vi "labview_robotjoint_states_Server.vi"() -> ()   [LabVIEW 2013]
doc: "Template server that runs individual ros topics, services, etc. This is cloned for each topic being run."
uses:
  SubVIs/_ROSControl.ctl
  SubVIs/_ROSDirection.ctl
  _ROSDefinition.vi
panel:
  out "Init Count":i32
  out "queue":string
  out "Connected":bool
  out "str to write":string
  out "Status":T1(ring) caption="Connected?"
  out "Specs":T3={"Server"="", "Node"="/labview", "Server Port"=5000, "URI (Subsc)"="", "Direction"=enum."Node"}
  out "Service Reply":string
  out "unregister":string="<?xml version='1.0'?>\n<methodResponse>\n<params>\n<param>\n<value><array><data>\n<value><int>1</int></value>\n<value><string>Registered [/labview] as publisher of [/robot/head/command_head_nod]</string></value>\n<value><array><data>\n<value><string>http://tuftsBaxter.local:56995/</string></value>\n</data></array></value>\n</data></array></value>\n</param>\n</params>\n</methodResponse>\n"
  out "Requests":T4(array[cluster])
  out "Last Reply":string
  in  "stop":bool
  out "error out":errorcluster
  out "Connections":T5(array[cluster])
  in  "Baxter":T6
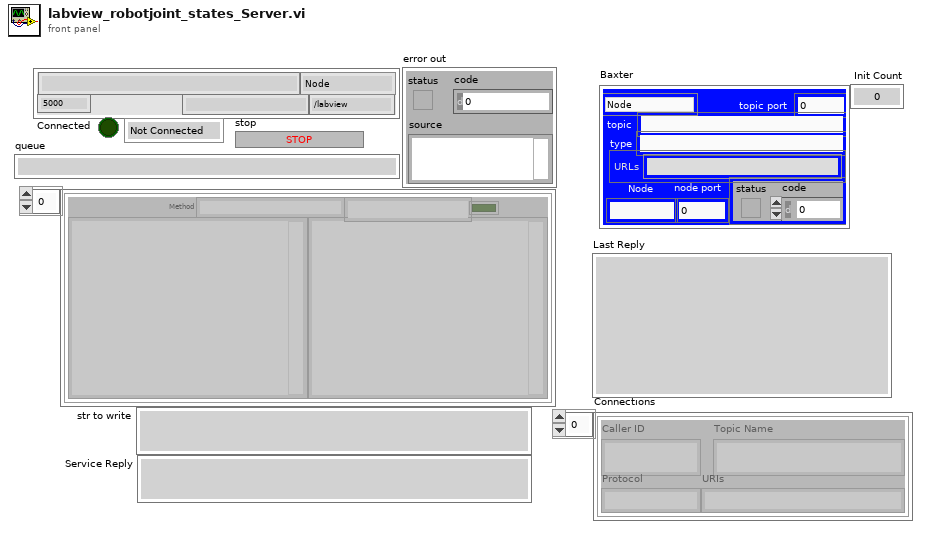
[diagram p1: front panel]
types:
  T1 = enum16{"Not Connected", "Registered", "Connected"}
  T2 = typedef "_ROSDirection.ctl" = enum16{"Node", "Publisher", "Subscriber", "Service Client"}
  T3 = cluster{"Server":string, "Node":string, "Server Port":u32, "URI (Subsc)":string, "Direction":T2}
  T4 = cluster{"First":string, "Second":string, "Method":string, "success":bool, "Dir1":string, "Dir2":string, "time":string}[]
  T5 = cluster{"Caller ID":string, "Topic Name":string, "Protocol":string, "URIs":string}[]
  T6 = typedef "_ROSControl.ctl" = cluster{"topic port":u16, "Node":string, "topic":string, "type":string, "node port":u32, "error ":errorcluster, "Direction":T2, "APIs":string[]}
  T7 = cluster{"data out":string, "data out 2":string, "data out 3":string, "Success?":bool, "data out 4":string, "data out 5":string, "time":string}[]
  T8 = cluster{"Code":i32, "Status Message":string, "APIs":string[]}
  T9 = cluster{"Server":string, "Node":string, "Server Port":u32, "URI (Subsc)":string, "connection":refnum<k5>, "Direction":T2}
  T10 = cluster{"Caller ID":string, "Topic Name":string, "Protocol":string, "URIs":string}
  T11 = cluster{string, "data out":string, "Node":string, bool, string, string, "Current Time":string}
  T12 = cluster{string, string, string, bool, string, string, "Current Time":string}
  T13 = cluster{"Protocol":string, "Code":i32, "IP":string, "Port":i32}
  T14 = cluster{"Node":string, "topic":string, "topic":string, "topic":string}
  T15 = cluster{"Code":i8, "statusMessage":string, "APIs":string[]}
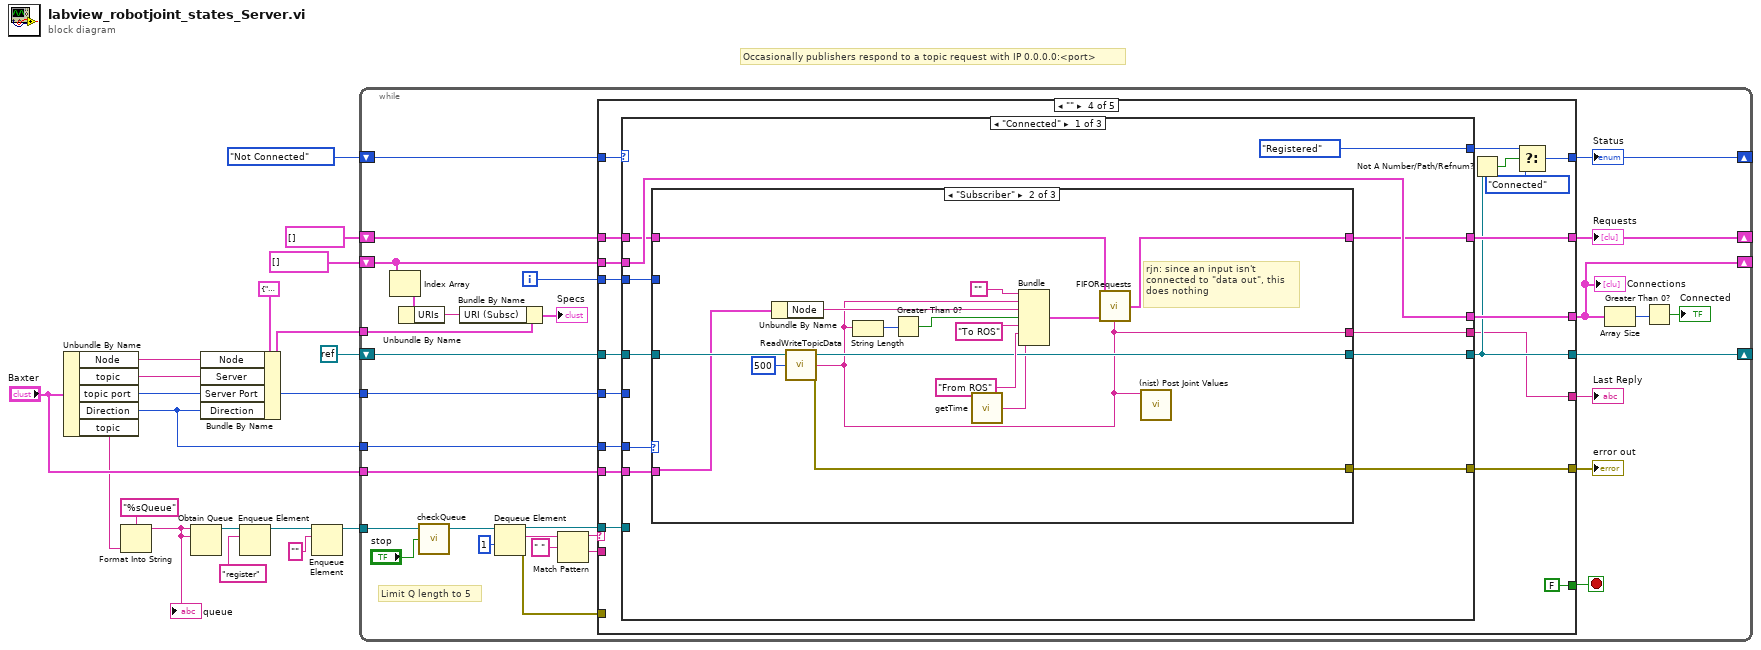
[diagram p0: block diagram]
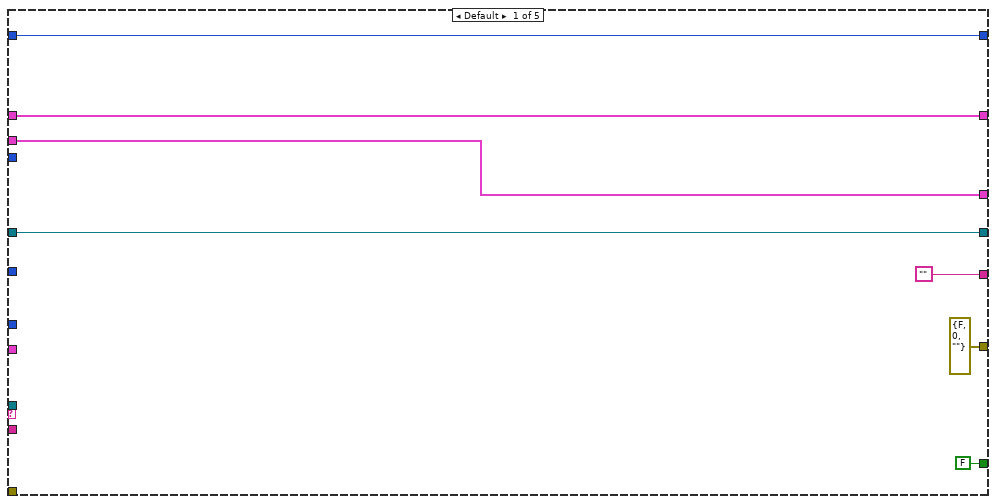
[diagram p2: hidden frame]
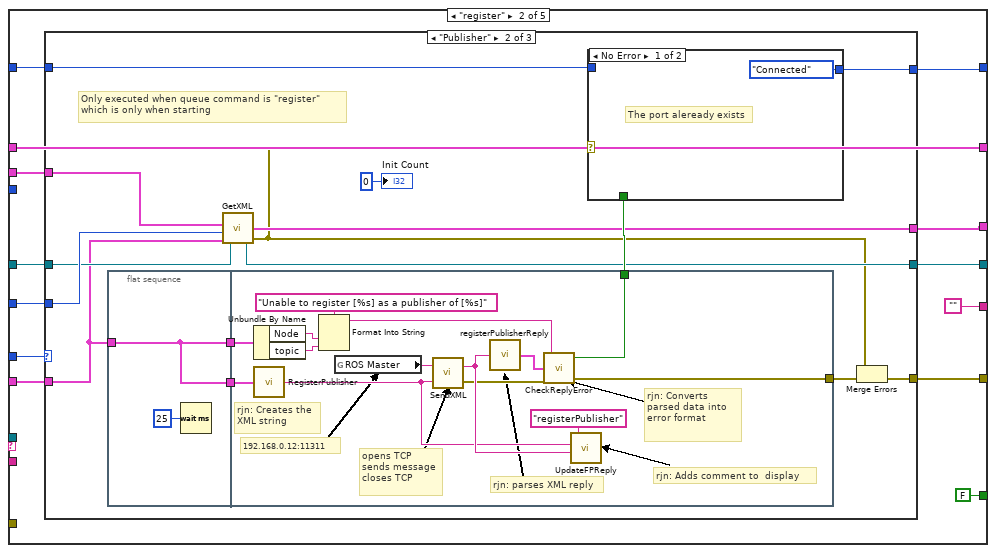
[diagram p3: hidden frame]
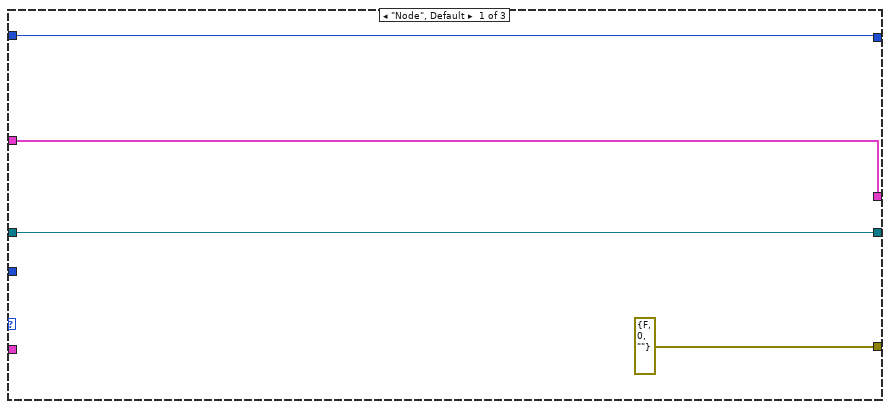
[diagram p4: hidden frame]
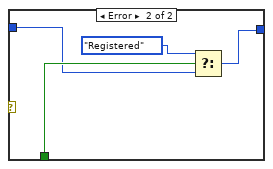
[diagram p5: hidden frame]
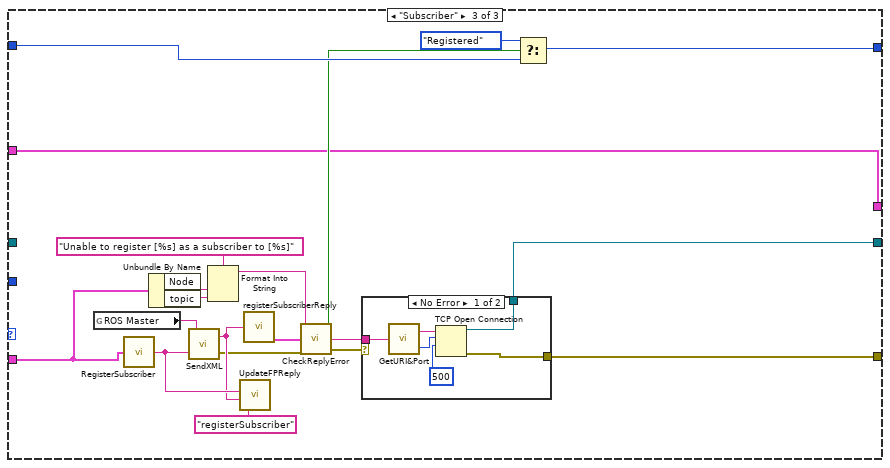
[diagram p6: hidden frame]
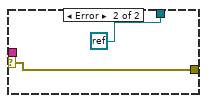
[diagram p7: hidden frame]
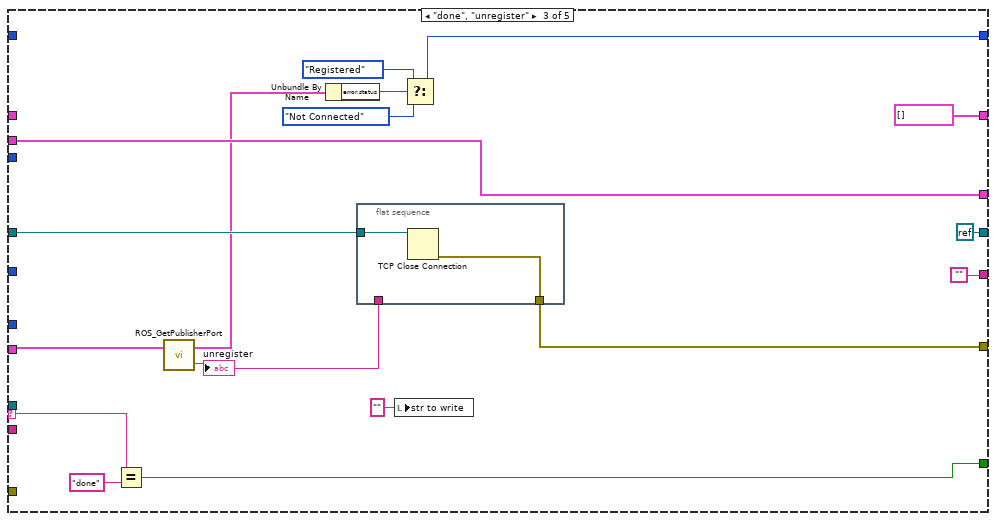
[diagram p8: hidden frame]
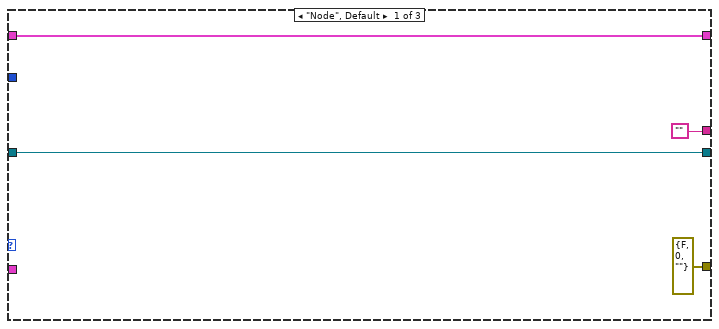
[diagram p9: hidden frame]
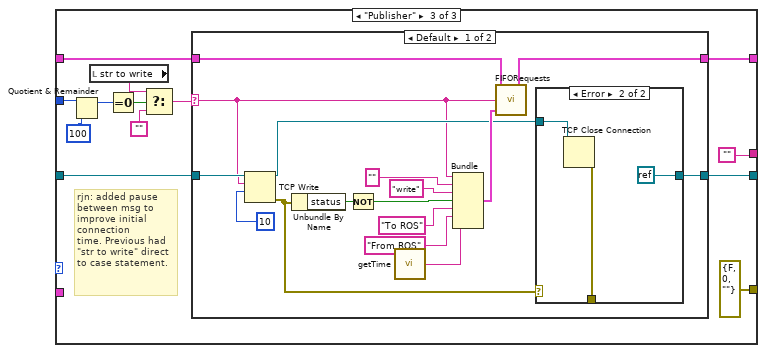
[diagram p10: hidden frame]
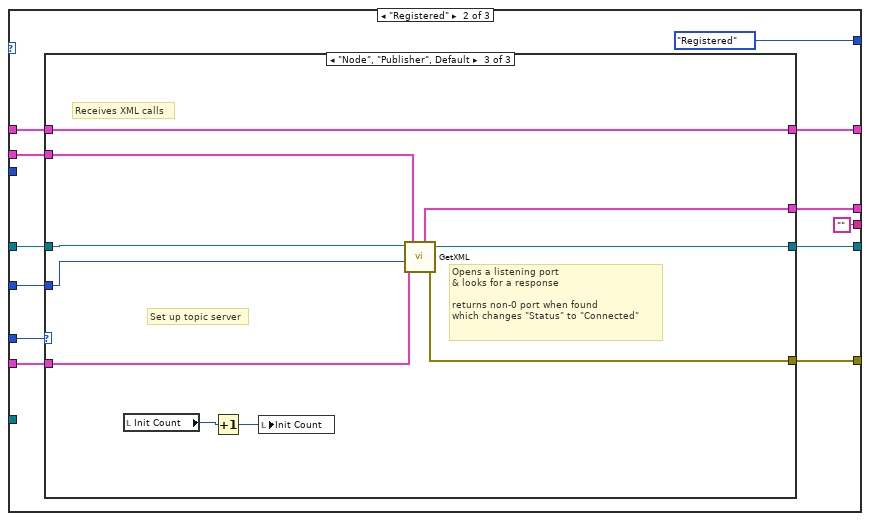
[diagram p13: hidden frame]
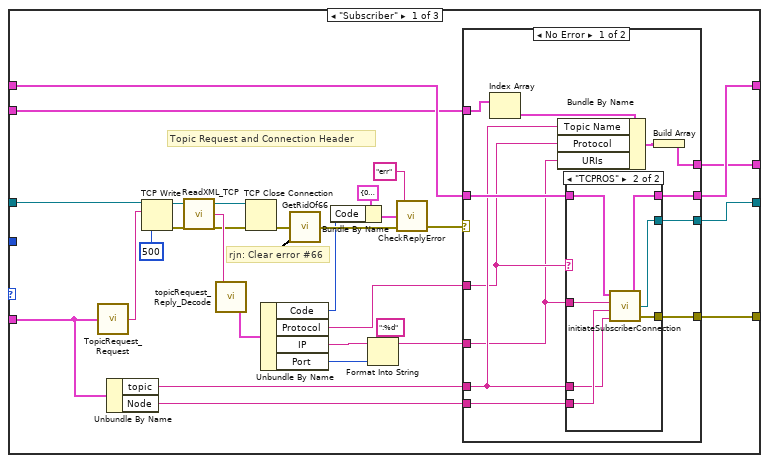
[diagram p14: hidden frame]
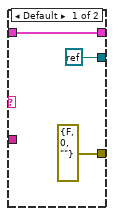
[diagram p15: hidden frame]
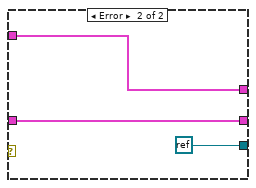
[diagram p16: hidden frame]
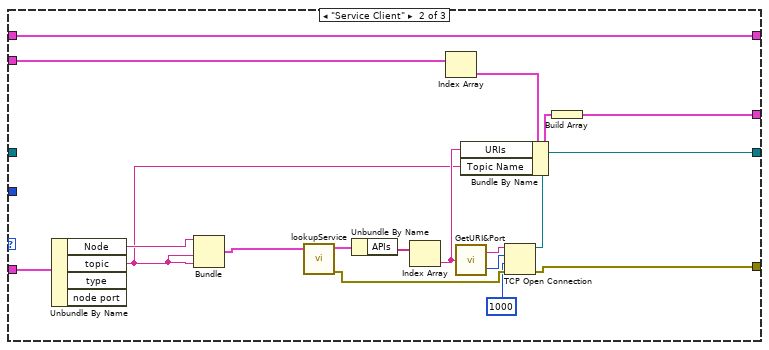
[diagram p17: hidden frame]
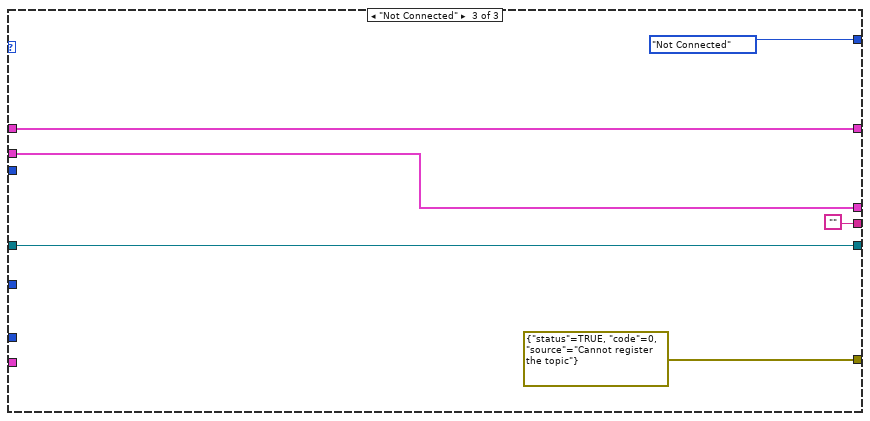
[diagram p18: hidden frame]
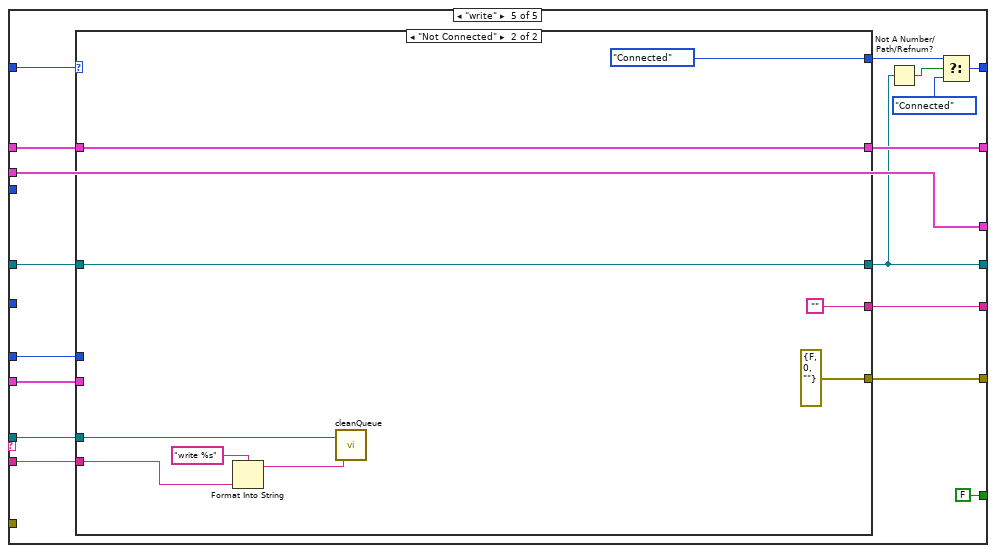
[diagram p19: hidden frame]
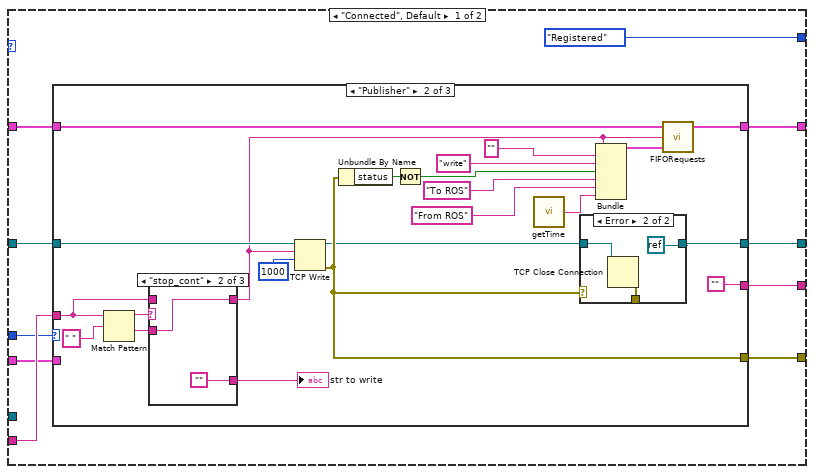
[diagram p20: hidden frame]
diagram:
  # "Occasionally publishers respond to a topic request with IP 0.0.0.0:<port>"
  n1 = Unbundle By Name("Baxter") -> ("Node"=w4:string, "topic"=w3:string, "topic port"=w1:u16, "Direction"=w2:T2, "topic"=w9:string)
  n2 = Format Into String(format string="%sQueue", w9) -> (resulting string=w18:string)  [unwired: 2 in, 1 out]
  "queue" <- w18
  n3 = Obtain Queue(name (unnamed)=w18, element data type=w18) -> (queue out=w12:refnum<queue>)  [unwired: 3 in, 2 out]
  n4 = Bundle By Name(cluster=T3 {"Server"="", "Node"="/labview", "Server Port"=5000, "URI (Subsc)"="", "Direction"=enum."Node"} ("Specs"), "Node"=w4, "Server"=w3, "Server Port"=w1, "Direction"=w2) -> (w10:T3)
  n5 = Enqueue Element(queue=w12, element="register") -> (queue out=w7:refnum<queue>)  [unwired: 2 in, 2 out]
  n6 = Enqueue Element(queue=w7, element="") -> (queue out=w6:refnum<queue>)  [unwired: 2 in, 2 out]
  n7 = while {
    tunnel: w1 -> [w50]
    shift-right: [w25] -> _
    shift-left: T5 [] ("Connections") -> [w34]
    shift-right: [w39] -> _
    shift-left: refnum<k0> refnum -> [w48]
    tunnel: w2 -> [w49]
    tunnel: "Baxter" -> [w47]
    shift-right: [w40] -> _
    shift-left: T7 [] ("Requests In") -> [w41]
    shift-right: [w36] -> _
    shift-left: T1."Not Connected" ("Status") -> [w37]
    tunnel: w10 -> [w32]
    tunnel: w6 -> [w26]
    i -> [w21]
    stop <- w38 stop-if-true
    # "Limit Q length to 5"
    n8 = Index Array(array=w34) -> (element=w33:T10)  [unwired: 1 in]
    n9 = Unbundle By Name(w33) -> ("URIs"=w31:string)
    n10 = call "checkQueue.vi"("stop"="stop", "queue in"=w26) -> ("queue out"=w28:refnum<queue>)  [unwired: 3 in]
    n11 = Bundle By Name(cluster=w32, "URI (Subsc)"=w31) -> (→"Specs":T3)
    n12 = Dequeue Element(queue=w28, timeout in ms (-1)=1) -> (queue out=w29:refnum<queue>, element=w45:string, error out=w22:errorcluster)  [unwired: 1 in, 1 out]
    n13 = Match Pattern(string=w45, regular expression=" ") -> (before substring=w43:string, after substring=w42:string)  [unwired: 1 in, 2 out]
    n14 = case shown="\"\"" w43 {
      selector: w43 -> [_ _ w144 _ _]
      tunnel: w50 -> [_ w69 _ w176 _]
      tunnel: w34 -> [w57 w61 w154 w175 w360]
      tunnel: [w57 w60 w154 w174 w360] -> w25
      tunnel: w49 -> [_ w70 _ w173 w352]
      tunnel: [w56 w66 refnum<k0> refnum w167 w353] -> w39
      tunnel: w48 -> [w56 w65 w155 w168 w359]
      tunnel: w47 -> [_ w68 w153 w172 w350]
      tunnel: w42 -> [_ _ _ _ w357]
      tunnel: [FALSE FALSE w142 FALSE FALSE] -> w38
      tunnel: [errorcluster {"status"=FALSE, "code"=0, "source"=""} ("error out") w67 w147 w169 w354] -> w35
      tunnel: w41 -> [w55 w64 _ w171 w356]
      tunnel: [w55 w64 T7 [] ("Requests Out") w170 w355] -> w40
      tunnel: w37 -> [w54 w63 _ w161 w358]
      tunnel: [w54 w62 w149 w162 w345] -> w36
      tunnel: ["" "" "" w166 w351] -> w20
      tunnel: w29 -> [_ _ _ w165 w349]
      tunnel: w22 -> [_ _ _ _ _]
      tunnel: w21 -> [_ _ _ w158 _]
      frame Default {
      }
      frame "register" {
        n15 = case shown="\"Publisher\"" w70 {
          tunnel: w69 -> [_ w84 _]
          tunnel: w68 -> [_ w81 w121]
          tunnel: [errorcluster {"status"=FALSE, "code"=0, "source"=""} ("error IO") w79 w118] -> w67
          tunnel: [w74 w82 w119] -> w66
          tunnel: w65 -> [w74 w83 _]
          tunnel: w63 -> [w73 w88 w114]
          tunnel: [w73 w87 w112] -> w62
          tunnel: w61 -> [w72 w86 w111]
          tunnel: [w72 w85 w111] -> w60
          frame "Node", Default {
          }
          frame "Publisher" {
            # "Only executed when queue command is \"register\"\nwhich is only when starting"
            n16 = flat-sequence {
              tunnel: w81 -> [w90]
              tunnel: [w90] -> w77
              tunnel: [w90] -> w75
              tunnel: [w95] -> w89
              tunnel: [w93] -> w80
              tunnel: w77 -> [w94]
              tunnel: w75 -> [w92]
              frame #0 {
                n17 = Wait (ms)(milliseconds to wait=u32 25) -> ()  [unwired: 1 out]
              }
              frame #1 {
                # "rjn: Adds comment to  display"
                # "rjn: Converts parsed data into\nerror format"
                # "rjn: parses XML reply"
                # "192.168.0.12:11311"
                # "opens TCP\nsends message\ncloses TCP"
                # "rjn: Creates the \nXML string"
                n18 = Unbundle By Name(w94) -> ("Node"=w101:string, "topic"=w100:string)
                n19 = call "RegisterPublisher.vi"("ROS"=w92) -> ("XML"=w99:string)
                n20 = Format Into String(format string="Unable to register [%s] as a publisher of [%s]", w101, w100) -> (resulting string=w97:string)  [unwired: 2 in, 1 out]
                n21 = global read "_ROSDefinition.vi" "ROS Master"() -> (w105:string)
                n22 = call "SendXML.vi"("Send"=w99, "URI in"=w105) -> ("error out"=w96:errorcluster, "Reply"=w104:string)
                n23 = call "registerPublisherReply.vi"("Response"=w104) -> ("Response"=w98:T8)
                n24 = call "CheckReplyError.vi"("error in"=w96, "Response"=w98, "Error String"=w97) -> ("error out"=w93:errorcluster, "Registered?"=w95:bool)  [unwired: 1 out]
                n25 = call "UpdateFPReply.vi"("Reply"=w104, "Sent"=w99, "method"="registerPublisher") -> ()  [unwired: 3 in]
              }
            }
            n26 = call "GetXML.vi"("Baxter"=w81, "topic port"=w84, "Connections"=w86, "connection ID in"=w83) -> ("error IO"=w78:errorcluster, "Subscribers"=w85:T5, "connection ID out"=w82:refnum<k5>)
            n27 = case shown="No Error" w78 {
              tunnel: w89 -> [_ w110]
              tunnel: w88 -> [_ w109]
              tunnel: [T1."Connected" ("f") w107] -> w87
              frame No Error {
                # "The port aleready exists"
              }
              frame Error {
                n28 = Select(t=T1."Registered", s=w110, f=w109) -> (s? t:f=w107:T1)
              }
            }
            n29 = Merge Errors(w78, w80) -> (w79:errorcluster)
            "Init Count" <- 0
          }
          frame "Subscriber" {
            n30 = global read "_ROSDefinition.vi" "ROS Master"() -> (w130:string)
            n31 = call "RegisterSubscriber.vi"("ROS"=w121) -> ("XML"=w128:string)
            n32 = Unbundle By Name(w121) -> ("Node"=w125:string, "topic"=w124:string)
            n33 = call "SendXML.vi"("Send"=w128, "URI in"=w130) -> ("error out"=w117:errorcluster, "Reply"=w127:string)
            n34 = Format Into String(format string="Unable to register [%s] as a subscriber to [%s]", w125, w124) -> (resulting string=w122:string)  [unwired: 2 in, 1 out]
            n35 = call "UpdateFPReply.vi"("Reply"=w127, "Sent"=w128, "method"="registerSubscriber") -> ()  [unwired: 3 in]
            n36 = call "registerSubscriberReply.vi"("Response"=w127) -> ("Response"=w126:T8)
            n37 = call "CheckReplyError.vi"("error in"=w117, "Response"=w126, "Error String"=w122) -> ("error out"=w116:errorcluster, "URI"=w120:string, "Registered?"=w113:bool)
            n38 = case shown="No Error" w116 {
              selector: w116 -> [_ w138]
              tunnel: w120 -> [w136 _]
              tunnel: [w132 refnum<k0> refnum] -> w119
              tunnel: [w131 w138] -> w118
              frame No Error {
                n39 = call "GetURI&Port.vi"("URI in"=w136) -> ("Port"=w134:u16, "URI"=w135:string)
                n40 = TCP Open Connection(address=w135, remote port or service name=w134, timeout ms (60000)=500) -> (connection ID=w132:refnum<k5>, error out=w131:errorcluster)  [unwired: 2 in]
              }
              frame Error {
              }
            }
            n41 = Select(t=T1."Registered", s=w113, f=w114) -> (s? t:f=w112:T1)
          }
        }
      }
      frame "done", "unregister" {
        n42 = Equal?(x=w144, y="done") -> (x = y?=w142:bool)
        n43 = call "ROS_GetPublisherPort.vi"("ROS in"=w153) -> ("Response"=w145:string, "ROS out"=w152:T6)  [unwired: 1 in]
        "unregister" <- w145
        n44 = Unbundle By Name(w152) -> ("error.status"=w148:bool)
        n45 = flat-sequence {
          tunnel: w155 -> [w157]
          tunnel: [w156] -> w147
          tunnel: w145 -> [_]
          frame #0 {
            n46 = TCP Close Connection(connection ID=w157) -> (error out=w156:errorcluster)  [unwired: 2 in, 1 out]
          }
        }
        n47 = local write "str to write"("" ("str to write")) -> ()
        n48 = Select(t=T1."Registered" ("Status"), s=w148, f=T1."Not Connected") -> (s? t:f=w149:T1)
      }
      frame "" {
        n49 = case shown="\"Connected\"" w161 {
          tunnel: w176 -> [_ w254 _]
          tunnel: w175 -> [w186 w253 w342]
          tunnel: [w186 w252 w342] -> w174
          tunnel: w173 -> [w187 w251 _]
          tunnel: [w180 w250 w341] -> w167
          tunnel: w168 -> [w185 w249 w341]
          tunnel: w172 -> [w184 w248 _]
          tunnel: w171 -> [w183 w247 w343]
          tunnel: [w182 w246 w343] -> w170
          tunnel: [w181 w245 errorcluster {"status"=TRUE, "code"=0, "source"="Cannot register the topic"} ("error out")] -> w169
          tunnel: [w179 "" ""] -> w166
          tunnel: w165 -> [_ _ _]
          tunnel: [T1."Registered" ("f") T1."Registered" ("f") T1."Not Connected" ("f")] -> w160
          tunnel: w158 -> [w177 _ _]
          frame "Connected" {
            n50 = case shown="\"Subscriber\"" w187 {
              tunnel: w185 -> [w190 w207 w218]
              tunnel: w184 -> [_ w200 _]
              tunnel: w183 -> [w191 w205 w220]
              tunnel: [w191 w204 w219] -> w182
              tunnel: [errorcluster {"status"=FALSE, "code"=0, "source"=""} ("error out") w203 errorcluster {"status"=FALSE, "code"=0, "source"=""} ("error out")] -> w181
              tunnel: [w190 w194 w217] -> w180
              tunnel: ["" w192 ""] -> w179
              tunnel: w177 -> [_ _ w214]
              frame "Node", Default {
              }
              frame "Subscriber" {
                # "rjn: since an input isn't\nconnected to \"data out\", this\ndoes nothing"
                n51 = Unbundle By Name(w200) -> ("Node"=w199:string)
                n52 = call "ReadWriteTopicData.vi"("timeout ms (1000)"=500, "connection ID in"=w207) -> ("error out"=w203:errorcluster, "data out"=w192:string, "connection ID out"=w194:refnum<k5>)  [unwired: 1 in]
                n53 = String Length(string=w192) -> (length=w202:i32)
                n54 = Greater Than 0?(x=w202) -> (x > 0?=w198:bool)
                n55 = call "getTime.vi"() -> ("Current Time"=w193:string)  [unwired: 1 in]
                n56 = Bundle("", "data out"=w192, "Node"=w199, w198, "To ROS", "From ROS", "Current Time"=w193) -> (w195:T11)  [unwired: 1 in]
                n57 = call "FIFORequests.vi"("New One"=w195, "data out"=w192, "Requests In"=w205) -> ("Requests Out"=w204:T7)
                n58 = call "(nist) Post Joint Values.vi"("Reply"=w192) -> ()  [unwired: 11 in]
              }
              frame "Publisher" {
                # "rjn: added pause \nbetween msg to \nimprove initial\nconnection\ntime. Previous had\n\"str to write\" direct\nto case statement."
                n59 = Quotient & Remainder(x=w214, y=100) -> (x-y*floor(x/y)=w212:i32)  [unwired: 1 out]
                n60 = local read "str to write"() -> (w210:string)
                n61 = Equal To 0?(x=w212) -> (x = 0?=w211:bool)
                n62 = Select(t=w210, s=w211, f="") -> (s? t:f=w208:string)
                n63 = case shown="Default" w208 {
                  selector: w208 -> [w221 _]
                  tunnel: w220 -> [w229 w242]
                  tunnel: [w228 w242] -> w219
                  tunnel: w218 -> [w226 w241]
                  tunnel: [w225 w241] -> w217
                  frame Default {
                    n64 = TCP Write(connection ID=w226, data in=w221, 9:10 ("timeout ms (25000)")) -> (connection ID out=w230:refnum<k5>, error out=w224:errorcluster)  [unwired: 1 in, 1 out]
                    n65 = Unbundle By Name(w224) -> ("status"=w232:bool)
                    n66 = Not(x=w232) -> (.not. x?=w231:bool)
                    n67 = call "getTime.vi"() -> ("Current Time"=w222:string)  [unwired: 1 in]
                    n68 = Bundle(w221, "", "write", w231, "To ROS", "From ROS", "Current Time"=w222) -> (w233:T12)  [unwired: 1 in]
                    n69 = call "FIFORequests.vi"("New One"=w233, "data out"=w221, "Requests In"=w229) -> ("Requests Out"=w228:T7)
                    n70 = case shown="Error" w224 {
                      tunnel: w230 -> [w237 w240]
                      tunnel: [w237 refnum<k0> refnum] -> w225
                      tunnel: [_ w238] -> _
                      frame No Error {
                      }
                      frame Error {
                        n71 = TCP Close Connection(connection ID=w240) -> (error out=w238:errorcluster)  [unwired: 2 in, 1 out]
                      }
                    }
                  }
                  frame "" {
                  }
                }
              }
            }
          }
          frame "Registered" {
            n72 = case shown="\"Node\", \"Publisher\", Default" w251 {
              tunnel: w254 -> [_ _ w330]
              tunnel: w253 -> [w264 w315 w337]
              tunnel: [w263 w313 w336] -> w252
              tunnel: [w267 w319 w335] -> w250
              tunnel: w249 -> [w284 _ w331]
              tunnel: w248 -> [w272 w326 w334]
              tunnel: w247 -> [w270 w327 w333]
              tunnel: [w269 w327 w333] -> w246
              tunnel: [w268 w318 w332] -> w245
              frame "Subscriber" {
                # "rjn: Clear error #66"
                # "Topic Request and Connection Header"
                n73 = call "TopicRequest_Request.vi"("ROS"=w272) -> ("XML"=w283:string)
                n74 = Unbundle By Name(w272) -> ("topic"=w255:string, "Node"=w271:string)
                n75 = TCP Write(connection ID=w284, data in=w283, 9:500 ("timeout ms (25000)")) -> (connection ID out=w282:refnum<k5>, error out=w281:errorcluster)  [unwired: 1 in, 1 out]
                n76 = call "ReadXML_TCP.vi"("error in"=w281, "connection ID in"=w282) -> ("error out"=w277:errorcluster, "data out"=w279:string, "connection ID out"=w278:refnum<k5>)  [unwired: 1 in]
                n77 = call "topicRequest_Reply_Decode.vi"("Topic Request Reply"=w279) -> ("Topic Request Reply"=w276:T13)
                n78 = TCP Close Connection(connection ID=w278, error in (no error)=w277) -> (error out=w275:errorcluster)  [unwired: 1 in, 1 out]
                n79 = Unbundle By Name(w276) -> ("Code"=w258:i32, "Protocol"=w266:string, "IP"=w262:string, "Port"=w273:i32)
                n80 = call "GetRidOf66.vi"("error in (no error)"=w275) -> ("error out"=w260:errorcluster)
                n81 = Bundle By Name(cluster=T8 {"Code"=0, "Status Message"="", "APIs"=[]} ("Response"), "Code"=w258) -> (w256:T8)
                n82 = Format Into String(format string=":%d", initial string=w262, w273) -> (resulting string=w265:string)  [unwired: 1 in, 1 out]
                n83 = call "CheckReplyError.vi"("error in"=w260, "Response"=w256, "Error String"="err" ("source")) -> ("error out"=w259:errorcluster)  [unwired: 2 out]
                n84 = case shown="No Error" w259 {
                  tunnel: w266 -> [w288 _]
                  tunnel: w265 -> [w287 _]
                  tunnel: w271 -> [w296 _]
                  tunnel: w255 -> [w289 _]
                  tunnel: w270 -> [w295 w307]
                  tunnel: [w294 w307] -> w269
                  tunnel: [w293 _] -> w268
                  tunnel: [w292 refnum<k0> refnum] -> w267
                  tunnel: w264 -> [w291 w308]
                  tunnel: [w285 w308] -> w263
                  frame No Error {
                    n85 = Index Array(array=w291) -> (element=w290:T10)  [unwired: 1 in]
                    n86 = Bundle By Name(cluster=w290, "Topic Name"=w289, "Protocol"=w288, "URIs"=w287) -> (w286:T10)
                    n87 = case shown="\"TCPROS\"" w288 {
                      tunnel: w287 -> [_ w306]
                      tunnel: w296 -> [_ w305]
                      tunnel: w289 -> [_ w304]
                      tunnel: w295 -> [w298 w300]
                      tunnel: [w298 w303] -> w294
                      tunnel: [errorcluster {"status"=FALSE, "code"=0, "source"=""} ("error out") w302] -> w293
                      tunnel: [refnum<k0> refnum w301] -> w292
                      frame Default {
                      }
                      frame "TCPROS" {
                        n88 = call "initiateSubscriberConnection.vi"("topic"=w304, "Node"=w305, "URI"=w306, "Requests In"=w300) -> ("error out"=w302:errorcluster, "connection ID out"=w301:refnum<k5>, "Requests Out"=w303:T7)
                      }
                    }
                    n89 = Build Array(w286) -> (w285:T5)
                  }
                  frame Error {
                  }
                }
              }
              frame "Service Client" {
                n90 = Unbundle By Name(w326) -> ("Node"=w325:string, "topic"=w311:string)  [unwired: 2 out]
                n91 = Bundle("Node"=w325, "topic"=w311, "topic"=w311, "topic"=w311) -> (w324:T14)  [unwired: 1 in]
                n92 = call "lookupService.vi"("Parameters"=w324) -> ("Reply"=w323:T15, "error out"=w312:errorcluster)  [unwired: 4 in, 2 out]
                n93 = Unbundle By Name(w323) -> ("APIs"=w322:string[])
                n94 = Index Array(array=w322) -> (element=w316:string)  [unwired: 1 in]
                n95 = Index Array(array=w315) -> (element=w317:T10)  [unwired: 1 in]
                n96 = call "GetURI&Port.vi"("URI in"=w316) -> ("Port"=w320:u16, "URI"=w321:string)
                n97 = Bundle By Name(cluster=w317, "URIs"=w316, "Topic Name"=w311) -> (w314:T10)
                n98 = TCP Open Connection(address=w321, remote port or service name=w320, timeout ms (60000)=1000, error in (no error)=w312) -> (connection ID=w319:refnum<k5>, error out=w318:errorcluster)  [unwired: 1 in]
                n99 = Build Array(w314) -> (w313:T5)
              }
              frame "Node", "Publisher", Default {
                # "Opens a listening port\n& looks for a response\n\nreturns non-0 port when found\nwhich changes \"Status\" to \"Connected\""
                # "Set up topic server"
                # "Receives XML calls"
                n100 = local read "Init Count"() -> (w329:i32)
                n101 = Increment(x=w329) -> (x+1=w328:i32)
                n102 = local write "Init Count"(w328) -> ()
                n103 = call "GetXML.vi"("Baxter"=w334, "topic port"=w330, "Connections"=w337, "connection ID in"=w331) -> ("error IO"=w332:errorcluster, "Subscribers"=w336:T5, "connection ID out"=w335:refnum<k5>)
              }
            }
          }
          frame "Not Connected" {
          }
        }
        n104 = Not A Number/Path/Refnum?(number/path/refnum=w167) -> (NaN/Path/Refnum?=w163:bool)
        n105 = Select(t=w160, s=w163, f=T1."Connected") -> (s? t:f=w162:T1)
      }
      frame "write" {
        n106 = case shown="\"Not Connected\"" w358 {
          tunnel: w359 -> [w370 w429]
          tunnel: w357 -> [w367 w426]
          tunnel: w356 -> [w369 w430]
          tunnel: [w368 w430] -> w355
          tunnel: [w365 w429] -> w353
          tunnel: [w366 errorcluster {"status"=FALSE, "code"=0, "source"=""} ("error out")] -> w354
          tunnel: w352 -> [w364 _]
          tunnel: [w363 ""] -> w351
          tunnel: w350 -> [w362 _]
          tunnel: w349 -> [_ w428]
          tunnel: [T1."Registered" ("f") T1."Connected" ("f")] -> w346
          frame "Connected", Default {
            n107 = case shown="\"Publisher\"" w364 {
              tunnel: w370 -> [w373 w396 w412]
              tunnel: w369 -> [w374 w394 w421]
              tunnel: [w374 w393 w420] -> w368
              tunnel: w367 -> [_ w377 w419]
              tunnel: [errorcluster {"status"=FALSE, "code"=0, "source"=""} ("error out") w385 w418] -> w366
              tunnel: [w373 w383 refnum<k0> refnum] -> w365
              tunnel: ["" "" w417] -> w363
              tunnel: w362 -> [_ _ w416]
              frame "Node", Default {
              }
              frame "Publisher" {
                n108 = Match Pattern(string=w377, regular expression=" ") -> (before substring=w378:string, after substring=w379:string)  [unwired: 1 in, 2 out]
                n109 = case shown="\"stop_cont\"" w378 {
                  tunnel: w379 -> [_ w400 w401]
                  tunnel: [w397 w400 w401] -> w381
                  tunnel: ["" "" w401] -> w380
                  tunnel: w377 -> [w397 _ _]
                  frame Default {
                  }
                  frame "stop_cont" {
                  }
                  frame "cont" {
                  }
                }
                "str to write" <- w380
                n110 = TCP Write(connection ID=w396, data in=w381, 9:1000 ("timeout ms (25000)")) -> (connection ID out=w384:refnum<k5>, error out=w385:errorcluster)  [unwired: 1 in, 1 out]
                n111 = Unbundle By Name(w385) -> ("status"=w387:bool)
                n112 = Not(x=w387) -> (.not. x?=w386:bool)
                n113 = call "getTime.vi"() -> ("Current Time"=w376:string)  [unwired: 1 in]
                n114 = case shown="Error" w385 {
                  tunnel: w384 -> [w402 w405]
                  tunnel: [w402 refnum<k0> refnum] -> w383
                  tunnel: [_ w403] -> _
                  frame No Error {
                  }
                  frame Error {
                    n115 = TCP Close Connection(connection ID=w405) -> (error out=w403:errorcluster)  [unwired: 2 in, 1 out]
                  }
                }
                n116 = Bundle(w381, "", "write", w386, "To ROS", "From ROS", "Current Time"=w376) -> (w388:T12)  [unwired: 1 in]
                n117 = call "FIFORequests.vi"("New One"=w388, "data out"=w381, "Requests In"=w394) -> ("Requests Out"=w393:T7)
              }
              frame "Service Client" {
                n118 = Unbundle By Name(w416) -> ("topic"=w408:string, "Node"=w409:string, "APIs"=w414:string[], "Direction"=w407:T2)
                n119 = Index Array(array=w414) -> (element=w413:string)  [unwired: 1 in]
                n120 = local write "Service Reply"("" ("Service Reply")) -> ()
                n121 = Bundle By Name(cluster=T9 {"Server"="", "Node"="/labview", "Server Port"=5000, "URI (Subsc)"="", "connection"=refnum, "Direction"=enum."Node"} ("Specs"), "Server"=w408, "Node"=w409, "URI (Subsc)"=w413, "connection"=w412, "Direction"=w407) -> (w411:T9)
                n122 = call "ROS_Service_Setup.vi"("Specs"=w411, "Msg to Send"=w419, "Requests In"=w421) -> ("error out"=w418:errorcluster, "Reply"=w417:string, "Requests Out"=w420:T7)
                "Service Reply" <- w417
              }
            }
          }
          frame "Not Connected" {
            n123 = Format Into String(format string="write %s", w426) -> (resulting string=w425:string)  [unwired: 2 in, 1 out]
            n124 = call "cleanQueue.vi"("String"=w425, "queue in"=w428) -> ()  [unwired: 1 in, 1 out]
          }
        }
        n125 = Not A Number/Path/Refnum?(number/path/refnum=w353) -> (NaN/Path/Refnum?=w347:bool)
        n126 = Select(t=w346, s=w347, f=T1."Connected") -> (s? t:f=w345:T1)
      }
    }
    "error out" <- w35
    "Requests" <- w40
    "Status" <- w36
    "Connections" <- w25
    "Last Reply" <- w20
    n127 = Array Size(array=w25) -> (size(s)=w24:i32)
    n128 = Greater Than 0?(x=w24) -> (x > 0?=→"Connected":bool)
  }
